vi "BRig_dataExp_Cue2Switch_Prob_PreR.vi"() -> (2 "output_Cue2Switch_Prob_PreR":i32)   [LabVIEW 2014]
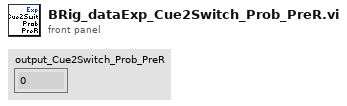
[diagram p1: front panel]
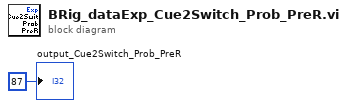
[diagram p0: block diagram]
diagram:
  "output_Cue2Switch_Prob_PreR" <- 87 ("output_iBlock")
